vi "Actor Core.vi"(8 "error in":errorcluster, 11 "BuildWorker in":refnum<class "BuildWorker.lvclass">) -> (0 "error out":errorcluster, 3 "Actor out":refnum<class "Actor.lvclass">)   [LabVIEW 2017, in "BuildWorker.lvlib" / "BuildWorker.lvclass"]
doc: "(<B>Filename</B>: Actor Framework.lvlib:Actor.lvclass:Actor Core.vi)\n\nReceives messages to the actor, reacts to them, and initiates any error handling that may shut the actor down.\n\nDescendant classes may override this VI to append parallel tasks for the actor to complete while it handles messages. Overrides use the Call Parent Method node."
uses:
  BuildWorker.lvclass
  Volumes/Data/Users/benji667/Git/BuildFarm/WebSocket Server/Actors/Actor wHelper/Actor wUI/Actor wUI.lvclass
  <vilib>/ActorFramework/Actor/Actor.lvclass
  BuildWorker.lvclass/BuildWorker.ctl
  WebSocket Server/Actors/Actor wHelper/Actor wUI/Actor wUI.lvclass/Actor wUI.ctl
  WebSocket Server/Actors/Actor wHelper/Actor wUI/Write UI Ref.vi
  WebSocket Server/Actors/Actor wHelper/Actor wUI/Actor wUI.lvclass
panel:
  out "BuildWorker Name":string
  out "BuildServer Port":u16
  in  "TaskList":i32(listbox)
  out "status":string
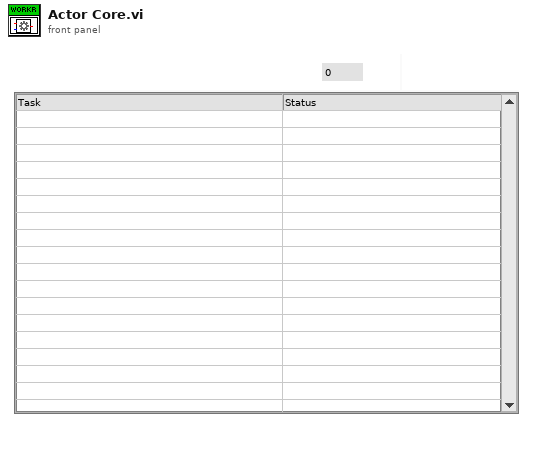
[diagram p1: front panel]
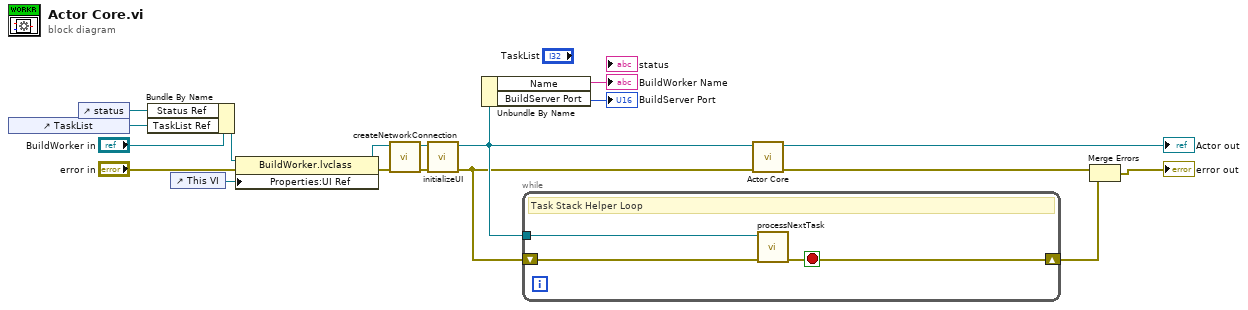
[diagram p0: block diagram]
diagram:
  n1 = control-ref of="TaskList"() -> (w12:refnum<vi>)
  n2 = control-ref of="status"() -> (w8:refnum<vi>)
  n3 = Bundle By Name(cluster="BuildWorker in", "Status Ref"=w8, "TaskList Ref"=w12) -> (w1:refnum<class "BuildWorker.lvclass">)
  n4 = control-ref of="This VI"() -> (w4:refnum<vi>)
  n5 = property class="BuildWorker.lvclass"(reference=w1, error in="error in", "Properties:UI Ref"=w4) -> (reference out=w7:refnum<class "BuildWorker.lvclass">, error out=w5:errorcluster)
  n6 = call "createNetworkConnection.vi"("error in (no error)"=w5, "BuildWorker in"=w7) -> ("error out"=w10:errorcluster, "BuildWorker out"=w3:refnum<class "BuildWorker.lvclass">)  [unwired: 8 in]
  n7 = call "initializeUI.vi"("error in (no error)"=w10, "BuildWorker in"=w3) -> ("error out"=w9:errorcluster, "BuildWorker out"=w11:refnum<class "BuildWorker.lvclass">)  [unwired: 8 in]
  n8 = Unbundle By Name(w11) -> ("Name"=→"BuildWorker Name":string, "BuildServer Port"=→"BuildServer Port":u16)
  n9 = while {
    tunnel: w11 -> [w21]
    shift-right: [w19] -> w15
    shift-left: w9 -> [w20]
    stop <- w19 stop-if-true
    # "Task Stack Helper Loop"
    n10 = call "processNextTask.vi"("error in (no error)"=w20, "BuildWorker in"=w21) -> ("error out"=w19:errorcluster)  [unwired: 8 in, 1 out]
  }
  n11 = call-parent "Actor Core.vi"("error in"=w9, "Actor in"=w11) -> ("error out"=w18:errorcluster, "Actor out"=→"Actor out":refnum<class "Actor.lvclass">)  [unwired: 8 in]
  n12 = Merge Errors(w18, w15) -> (→"error out":errorcluster)
